vi "Query Status.vi"(0 "VISA resource name":refnum<visa-resource-name>, 5 "Channel (0: Channel 1)":i32(ring) items=["Channel 1", "Channel 2"], 11 "error in (no error)":errorcluster) -> (4 "VISA resource name out":refnum<visa-resource-name>, 8 "Transition Status":i32(ring) items=["Busy"=0, "Idle"=1, "Wait For Transition Trigger"=2, "Wait For Transition Arm"=4], 10 "Acquire Status":i32(ring) items=["Busy"=0, "Idle"=1, "Wait For Acquire Trigger"=2, "Wait For Acquire Arm"=4], 15 "error out":errorcluster)   [LabVIEW 2023, in "Agilent B2900 Series.lvlib"]
doc: "Query current instrument status"
uses:
  Agilent B2900 Series.lvlib
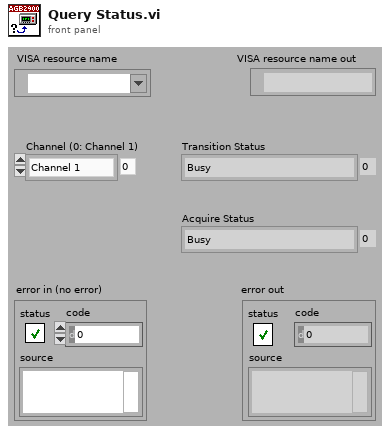
[diagram p1: front panel]
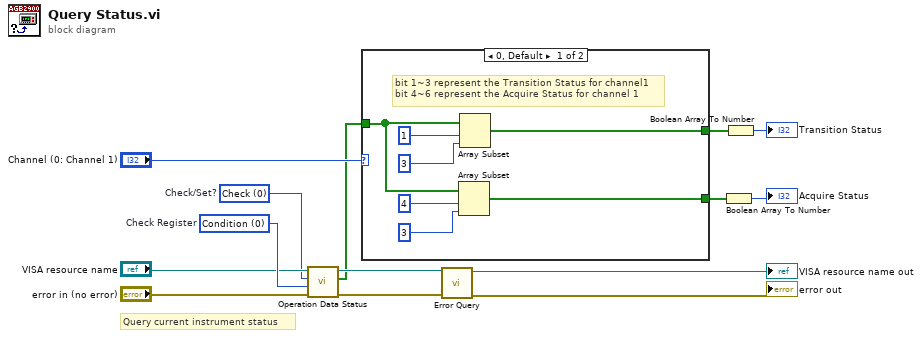
[diagram p0: block diagram]
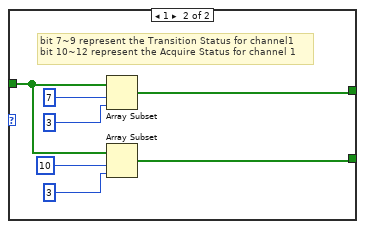
[diagram p2: hidden frame]
diagram:
  w1 = 0 items=["Check", "Set"]  # Check/Set?
  w7 = 0 items=["Condition", "Enable", "Event", "NTR", "PTR"]  # Check Register
  # "Query current instrument status"
  n1 = call "Operation Data Status.vi"("error in (no error)"="error in (no error)", "Operation Register To Check (0: Condition)"=w7, "Operation Mode (0: Check)"=w1, "VISA resource name"="VISA resource name") -> ("error out"=w3:errorcluster, "Operation Register Status"=w2:bool[], "VISA resource name out"=w4:refnum<visa-resource-name>)  [unwired: 5 in]
  n2 = case shown="0, Default" "Channel (0: Channel 1)" {
    tunnel: [w17 w28] -> w12
    tunnel: [w16 w23] -> w9
    tunnel: w2 -> [w15 w22]
    frame 0, Default {
      # "bit 1~3 represent the Transition Status for channel1\nbit 4~6 represent the Acquire Status for channel 1"
      n3 = Array Subset(array=w15, index=4, length=3) -> (w16:bool[])
      n4 = Array Subset(array=w15, index=1, length=3) -> (w17:bool[])
    }
    frame 1 {
      # "bit 7~9 represent the Transition Status for channel1\nbit 10~12 represent the Acquire Status for channel 1"
      n5 = Array Subset(array=w22, index=7, length=3) -> (w28:bool[])
      n6 = Array Subset(array=w22, index=10, length=3) -> (w23:bool[])
    }
  }
  n7 = call "Error Query.vi"("error in (no error)"=w3, "VISA resource name"=w4) -> ("error out"=→"error out":errorcluster, "VISA resource name out"=→"VISA resource name out":refnum<visa-resource-name>)  [unwired: 6 in, 2 out]
  n8 = Boolean Array To Number(Boolean array=w9) -> (number=→"Acquire Status":u32)
  n9 = Boolean Array To Number(Boolean array=w12) -> (number=→"Transition Status":u32)
